vi "FB_initialize.vi"() -> (0 "error out":errorcluster, 1 "Transformed Calibration Matrix":dbl[][](array[numeric]), 3 "FB out":refnum<k21>)   [LabVIEW 2021]
uses:
  <vilib>/DAQmx/create/channels.llb/DAQmx Create Channel (AI-Voltage-Basic).vi
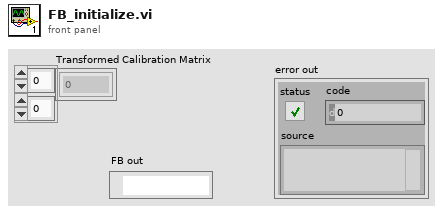
[diagram p1: front panel]
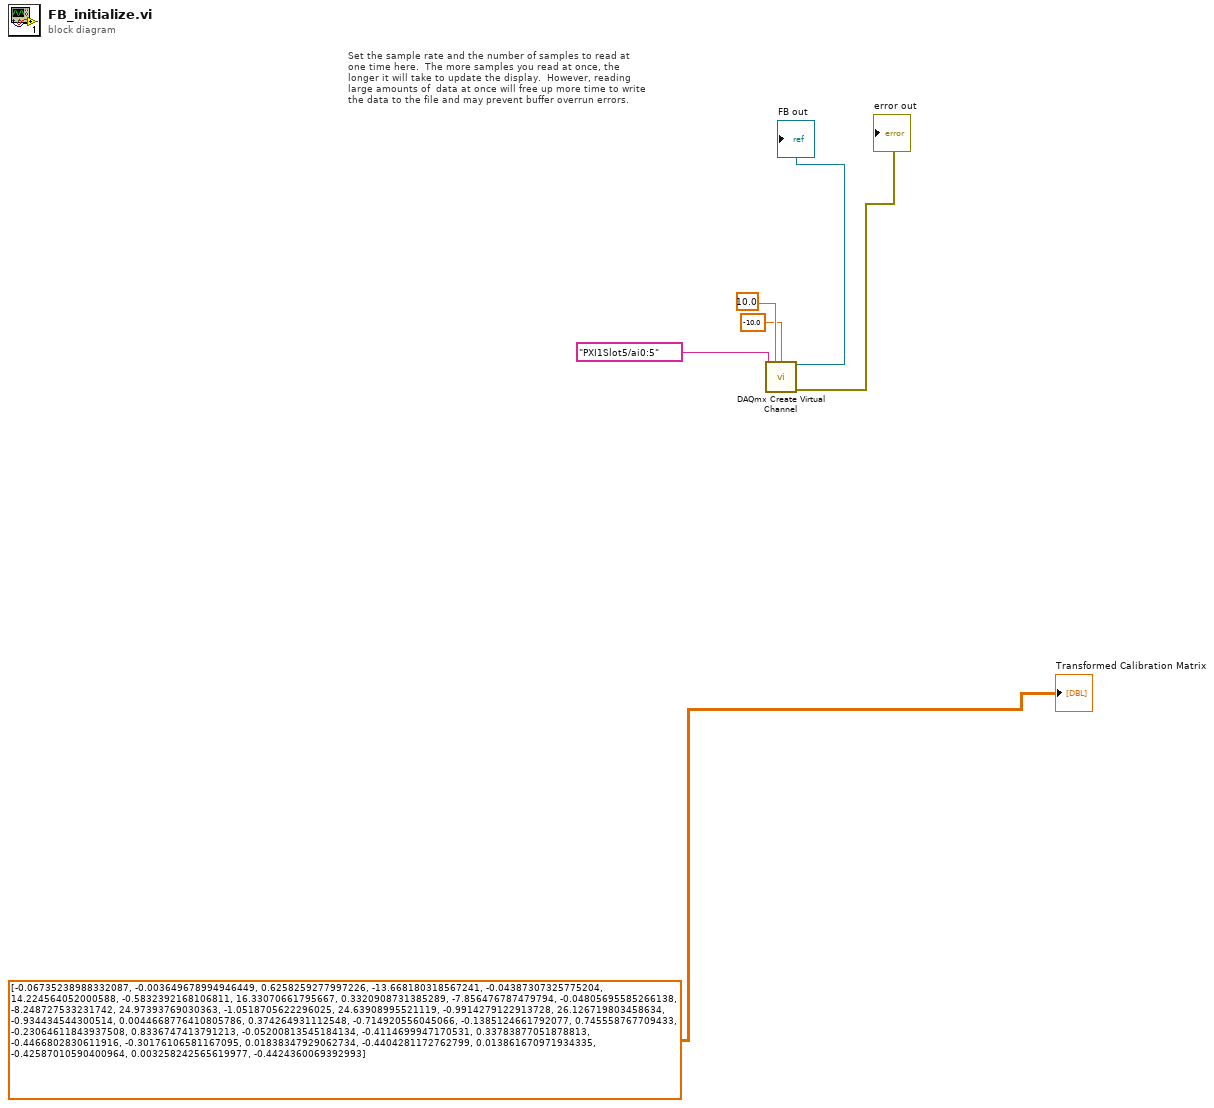
[diagram p0: block diagram]
diagram:
  # "Set the sample rate and the number of samples to read at\none time here.  The more samples you read at once, the\nlonger it will take to update the display.  However, reading\nlarge amounts of  data at once will free up more time to write\nthe data to the file and may prevent buffer overrun errors."
  n1 = call-poly <vilib>:"DAQmx Create Virtual Channel.vi"("maximum value"=10.0, "minimum value"=-10.0, "physical channels"=tag "PXI1Slot5/ai0:5") -> ("task out"=→"FB out":refnum<k21>, "error out"=→"error out":errorcluster)  [unwired: 11 in]
  "Transformed Calibration Matrix" <- dbl[][] [[-0.06735238988332087, -0.003649678994946449, 0.6258259277997226, -13.668180318567241, -0.04387307325775204, 14.224564052000588], [-0.5832392168106811, 16.33070661795667, 0.3320908731385289, -7.856476787479794, -0.04805695585266138, -8.248727533231742], [24.97393769030363, -1.0518705622296025, 24.63908995521119, -0.9914279122913728, 26.126719803458634, -0.934434544300514], [0.0044668776410805786, 0.374264931112548, -0.714920556045066, -0.1385124661792077, 0.745558767709433, -0.23064611843937508], [0.8336747413791213, -0.05200813545184134, -0.4114699947170531, 0.33783877051878813, -0.4466802830611916, -0.30176106581167095], [0.01838347929062734, -0.4404281172762799, 0.013861670971934335, -0.42587010590400964, 0.003258242565619977, -0.4424360069392993]] ("Calibration Matrix")
